vi "Algorithm.vi"(0 "LoadCall1":dbl, 1 "Wind available: 0 to 5 V DC":dbl, 3 "PV available: 0 to 5 V DC":dbl, 5 "LoadCall2":dbl, 9 "LoadCall3":dbl, 12 "Bus Voltage IN: -4 to 4 Vrms AC":dbl, 14 "Bus Current IN: -10 to 10 Vrms AC":dbl) -> (4 "LoadSw1":bool, 6 "LoadSw2":bool, 8 "LoadSw3":bool, 10 "Battery Discharge Sw":bool, 13 "Mains Request":sgl, 15 "Battery Charge Sw":bool)   [LabVIEW 2025]
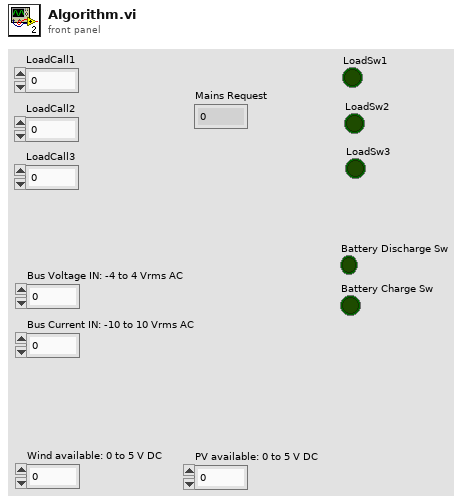
[diagram p1: front panel]
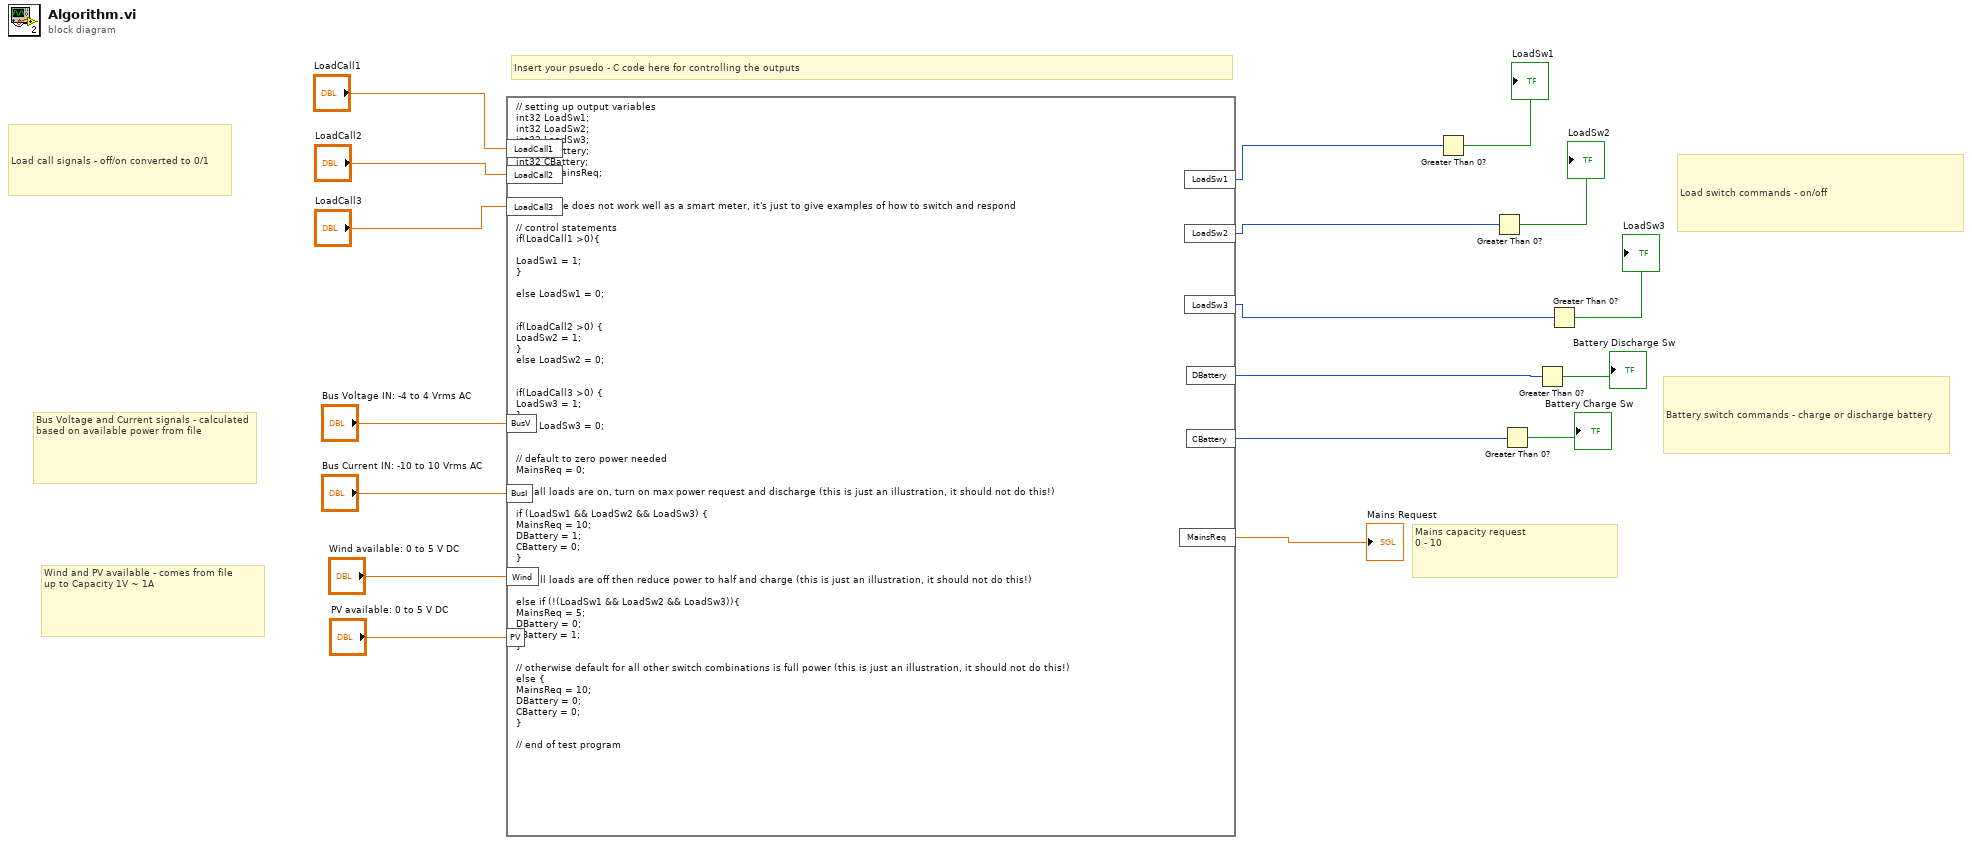
[diagram p0: block diagram]
diagram:
  # "Mains capacity request\n0 - 10"
  # "Battery switch commands - charge or discharge battery"
  # "Load switch commands - on/off"
  # "Wind and PV available - comes from file\nup to Capacity 1V ~ 1A"
  # "Bus Voltage and Current signals - calculated based on available power from file"
  # "Load call signals - off/on converted to 0/1"
  # "Insert your psuedo - C code here for controlling the outputs"
  n1 = formula code="// setting up output variables\nint32 LoadSw1; \nint32 LoadSw2;\nint32 LoadSw3;\nint32 DBattery;\nint32 CBattery;\nfloat32 MainsReq;\n\n\n// this code does not work well as a smart meter, it's just to give examples of how to switch and respond\n\n// control statements\nif(LoadCall1 >0){\n\nLoadSw1 = 1;\n}\n\nelse LoadSw1 = 0;\n\n\nif(LoadCall2 >0) {\nLoadSw2 = 1;\n}\nelse LoadSw2 = 0;\n\n\nif(LoadCall3 >0) {\nLoadSw3 = 1;\n}\nelse LoadSw3 = 0;\n\n\n// default to zero power needed\nMainsReq = 0;\n\n// if all loads are on, turn on max power request and discharge (this is just an illustration, it should not do this!)\n\nif (LoadSw1 && LoadSw2 && LoadSw3) {\nMainsReq = 10;\nDBattery = 1;\nCBattery = 0;\n}\n\n// if all loads are off then reduce power to half and charge (this is just an illustration, it should not do this!)\n\nelse if (!(LoadSw1 && LoadSw2 && LoadSw3)){\nMainsReq = 5;\nDBattery = 0;\nCBattery = 1;\n}\n\n// otherwise default for all other switch combinations is full power (this is just an illustration, it should not do this!)\nelse {\nMainsReq = 10;\nDBattery = 0;\nCBattery = 0;\n}\n\n// end of test program"("LoadCall1"="LoadCall1", "LoadCall2"="LoadCall2", "LoadCall3"="LoadCall3", "BusV"="Bus Voltage IN: -4 to 4 Vrms AC", "BusI"="Bus Current IN: -10 to 10 Vrms AC", "Wind"="Wind available: 0 to 5 V DC", "PV"="PV available: 0 to 5 V DC") -> ("LoadSw1"=w10:i32, "LoadSw2"=w7:i32, "DBattery"=w3:i32, "CBattery"=w1:i32, "LoadSw3"=w5:i32, "MainsReq"=→"Mains Request":sgl)
  n2 = Greater Than 0?(x=w10) -> (x > 0?=→"LoadSw1":bool)
  n3 = Greater Than 0?(x=w7) -> (x > 0?=→"LoadSw2":bool)
  n4 = Greater Than 0?(x=w1) -> (x > 0?=→"Battery Charge Sw":bool)
  n5 = Greater Than 0?(x=w3) -> (x > 0?=→"Battery Discharge Sw":bool)
  n6 = Greater Than 0?(x=w5) -> (x > 0?=→"LoadSw3":bool)
